vi "HumanExecute.vi"(8 "error in (no error)":errorcluster) -> (0 "error out":errorcluster)   [LabVIEW 2025]
doc: "Execute for Human\n\ninput:\n error in (cluster)\n\noutput:\n error out (cluster)"
uses:
  <vilib>/Rock Robotics/WPI/Joystick/XBox Axes Indexer.ctl
  <vilib>/Rock Robotics/WPI/Joystick/XBox Buttons Indexer.ctl
  <vilib>/Rock Robotics/WPI/ThirdParty/JAS_Junk/TrajLib/MathUtil_ApplyDeadband.vi
  <vilib>/Rock Robotics/WPI/ThirdParty/JAS_Junk/TrajLib/VI/DigSeqLogic_Edge_On.vi
  HumanGlobal.vi
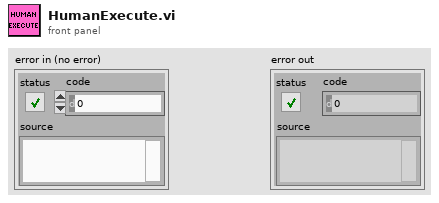
[diagram p1: front panel]
types:
  T1 = typedef "XBox Axes Indexer.ctl" = enum16{"Left X", "Left Y", "Left Trigger", "Right Trigger", "Right X", "Right Y"}
  T2 = typedef "XBox Buttons Indexer.ctl" = enum16{"A", "B", "X", "Y", "Left Bumper", "Right Bumper", "Back", "Start", "Left Joystick", "Right Joystick"}
  T3 = typedef "WPI_JoystickDevRef.ctl" = cluster{"Device":T4}
  T4 = typedef "WPI_JoystickDeviceEnum.ctl" = enum16{"USB 0", "USB 1", "USB 2", "USB 3", "USB 4", "USB 5"}
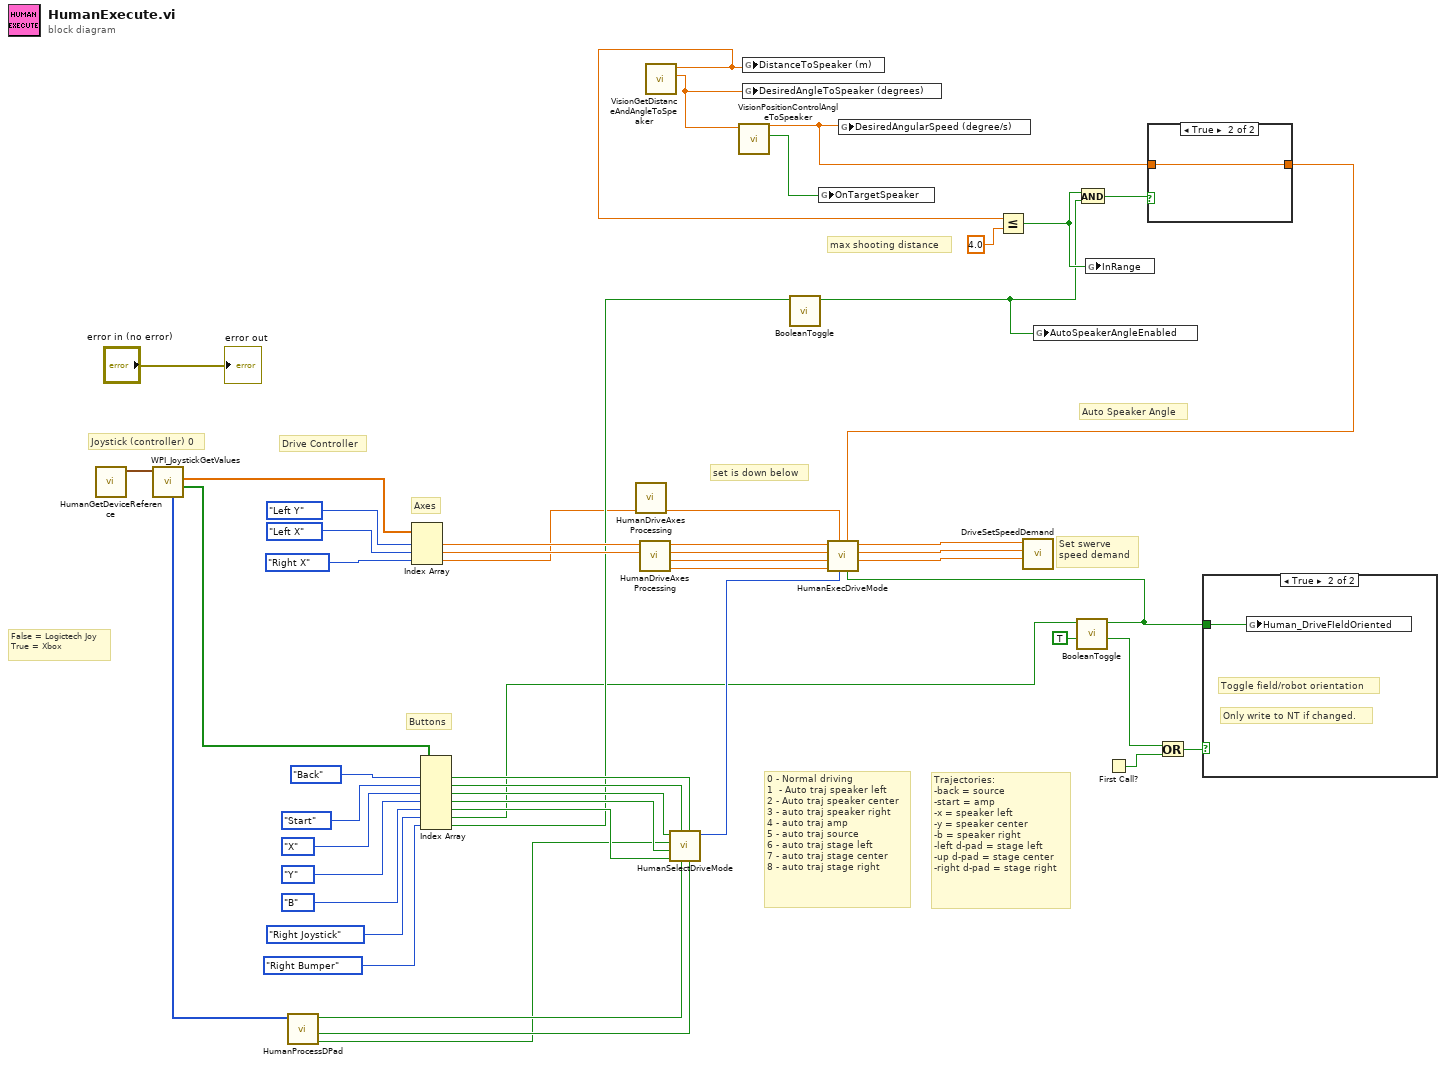
[diagram p0: block diagram]
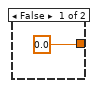
[diagram p3: hidden frame]
diagram:
  # "Auto Speaker Angle"
  # "0 - Normal driving\n1  - Auto traj speaker left \n2 - Auto traj speaker center\n3 - auto traj speaker right \n4 - auto traj amp\n5 - auto traj source\n6 - auto traj stage left\n7 - auto traj stage center\n8 - auto traj stage right"
  # "False = Logictech Joy\nTrue = Xbox"
  # "max shooting distance"
  # "Trajectories:\n-back = source\n-start = amp\n-x = speaker left\n-y = speaker center\n-b = speaker right\n-left d-pad = stage left\n-up d-pad = stage center\n-right d-pad = stage right"
  # "Buttons"
  # "Axes"
  # "set is down below"
  # "Set swerve\nspeed demand"
  # "Joystick (controller) 0"
  # "Drive Controller"
  n1 = call "HumanGetDeviceReference.vi"() -> ("Driver Joy"=w41:T3)  [unwired: 9 in, 2 out]
  n2 = call <vilib>:"WPI_JoystickGetValues.vi"("JoystickDevRef"=w41) -> ("Buttons"=w39:bool[], "Axes"=w40:dbl[], "POVs"=w50:i16[])  [unwired: 6 in, 2 out]
  n3 = call "HumanProcessDPad.vi"("POV"=w50) -> ("Right"=w26:bool, "Left"=w27:bool, "Up"=w28:bool)  [unwired: 7 in, 1 out]
  n4 = Index Array(array=w40, index #1=XBox_Axes_Indexer."Left Y" ("XBox Axes"), index #2=XBox_Axes_Indexer."Left X" ("XBox Axes"), index #3=XBox_Axes_Indexer."Right X" ("XBox Axes")) -> (element #1=w49:dbl, element #2=w48:dbl, element #3=w11:dbl)
  n5 = Index Array(array=w39, index #1=XBox_Buttons_Indexer."Back" ("Nothing"), index #2=XBox_Buttons_Indexer."Start" ("Nothing"), index #3=XBox_Buttons_Indexer."X" ("Nothing"), index #4=XBox_Buttons_Indexer."Y" ("Nothing"), index #5=XBox_Buttons_Indexer."B" ("Nothing"), index #6=XBox_Buttons_Indexer."Right Joystick" ("Nothing"), index #7=XBox_Buttons_Indexer."Right Bumper" ("Nothing")) -> (element #1=w33:bool, element #2=w32:bool, element #3=w31:bool, element #4=w30:bool, element #5=w29:bool, element #6=w4:bool, element #7=w15:bool)
  n6 = call "HumanDriveAxesProcessing.vi"("Right X"=w11) -> ("Right X"=w12:dbl)  [unwired: 7 in, 3 out]
  n7 = call "HumanDriveAxesProcessing.vi"("Left X"=w48, "Left Y"=w49) -> ("Right X"=w10:dbl, "Right Y"=w46:dbl, "Left X"=w47:dbl, "Left Y"=w45:dbl)  [unwired: 6 in]
  n8 = call "VisionGetDistanceAndAngleToSpeaker.vi"() -> ("DesiredAngle"=w23:dbl, "Distance"=w21:dbl)  [unwired: 10 in]
  n9 = call "HumanSelectDriveMode.vi"("AutoTrajStageLeft"=w27, "AutoTrajSource"=w33, "AutoTrajStageCenter"=w28, "AutoTrajAmp"=w32, "AutoTrajSpeakerRight"=w29, "AutoTrajSpeakerCenter"=w30, "AutoTrajStageRight"=w26, "AutoTrajSpeakerLeft"=w31) -> ("Drive Mode"=w25:i32)  [unwired: 3 in]
  n10 = call "VisionPositionControlAngleToSpeaker.vi"("TargetAngle"=w23) -> ("OnTargetSpeaker"=w22:bool, "DesiredAngularSpeed (degree/s)"=w19:dbl)  [unwired: 9 in]
  n11 = global write "HumanGlobal.vi" "DistanceToSpeaker (m)"(w21) -> ()
  n12 = global write "HumanGlobal.vi" "DesiredAngleToSpeaker (degrees)"(w23) -> ()
  n13 = call "BooleanToggle.vi"("Toggle Edge In"=w15) -> ("Output"=w14:bool)  [unwired: 9 in, 1 out]
  n14 = global write "HumanGlobal.vi" "OnTargetSpeaker"(w22) -> ()
  n15 = global write "HumanGlobal.vi" "DesiredAngularSpeed (degree/s)"(w19) -> ()
  n16 = Less Or Equal?(x=w21, y=4.0) -> (x <= y?=w18:bool)
  n17 = global write "HumanGlobal.vi" "AutoSpeakerAngleEnabled"(w14) -> ()
  n18 = call "BooleanToggle.vi"("InitialState"=TRUE, "Toggle Edge In"=w4) -> ("Changed"=w1:bool, "Output"=w3:bool)  [unwired: 8 in]
  n19 = And(x=w18, y=w14) -> (x .and. y?=w17:bool)
  n20 = global write "HumanGlobal.vi" "InRange"(w18) -> ()
  n21 = First Call?() -> (First Call?: T/F=w5:bool)
  n22 = case shown="True" w17 {
    tunnel: w19 -> [_ w53]
    tunnel: [0.0 w53] -> w13
    frame False {
    }
    frame True {
    }
  }
  n23 = call "HumanExecDriveMode.vi"("Enable Field Oriented Drive"=w3, "AutoSpeakerAngle"=w13, "State"=w25, "Rotation"=w12, "Right X"=w10, "Right Y"=w46, "Left X"=w47, "Left Y"=w45) -> ("AMotorDemand"=w44:dbl, "YMotorDemand"=w43:dbl, "XMotorDemand"=w42:dbl)  [unwired: 1 in]
  n24 = call "DriveSetSpeedDemand.vi"("ASpeedDemand (d/s)"=w44, "YSpeedDemand (ft/s)"=w43, "XSpeedDemand (ft/s)"=w42) -> ()  [unwired: 9 in]
  n25 = Or(x=w1, y=w5) -> (x .or. y?=w6:bool)
  n26 = case shown="True" w6 {
    tunnel: w3 -> [_ w54]
    frame False {
    }
    frame True {
      # "Only write to NT if changed."
      # "Toggle field/robot orientation"
      n27 = global write "HumanGlobal.vi" "Human_DriveFIeldOriented"(w54) -> ()
    }
  }
  "error out" <- "error in (no error)"
